vi "fgv_cursor_data.vi"(0 "cursor_idx_set":i32, 1 "plot_data_set":cluster{"array type (2D Dbl)":dbl[], dbl[]}[](array[cluster])=[{"array type (2D Dbl)"=array[301 elements], array[301 elements]}, {"array type (2D Dbl)"=array[301 elements], array[301 elements]}, {"array type (2D Dbl)"=array[301 elements], array[301 elements]}, {"array type (2D Dbl)"=array[301 elements], array[301 elements]}, {"array type (2D Dbl)"=[], []}, {"array type (2D Dbl)"=[], []}, {"array type (2D Dbl)"=[], []}, {"array type (2D Dbl)"=[], []}], 3 "cursor_mode_set":bool, 5 "cursor_pos_set":i32, 7 "cursor_color_set":T1, 9 "mode":string(combo)="Get", 11 "Error in":errorcluster, 12 "plot_id_set":i32) -> (4 "cursor_idx_get":i32, 6 "cursor_pos_get":i32, 8 "cursor_color_get":T1, 10 "cursor_data_get":T2, 13 "plot_id_get":i32, 14 "cursor_mode_get":bool, 15 "error out":errorcluster)   [LabVIEW 2025]
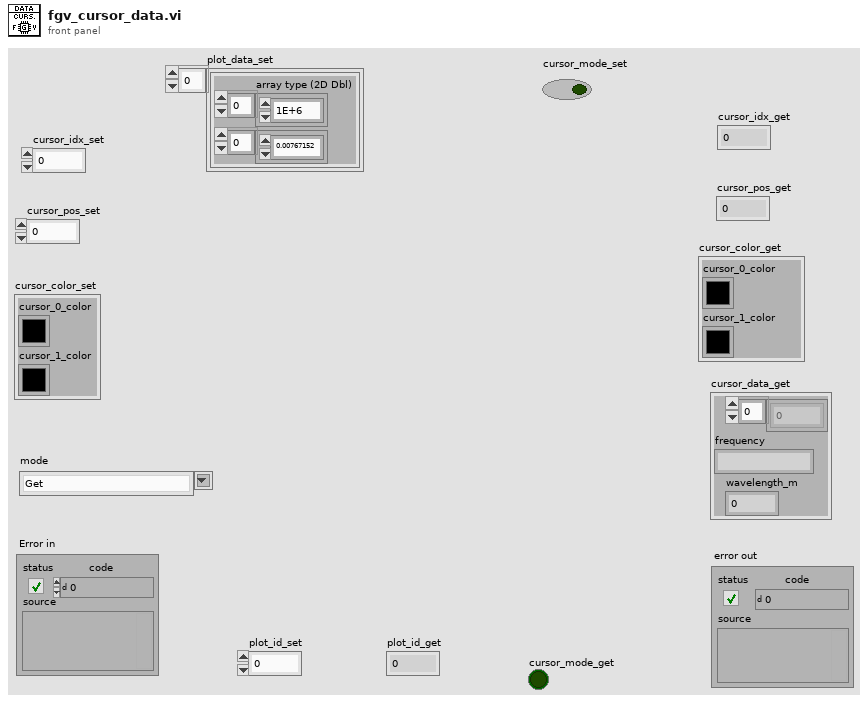
[diagram p1: front panel]
types:
  T1 = cluster{"cursor_0_color":u32, "cursor_1_color":u32}
  T2 = cluster{"cursor_data":dbl[], "frequency":string, "wavelength_m":dbl}
  T3 = cluster{dbl[], "String":string, "wavelength_m":dbl}
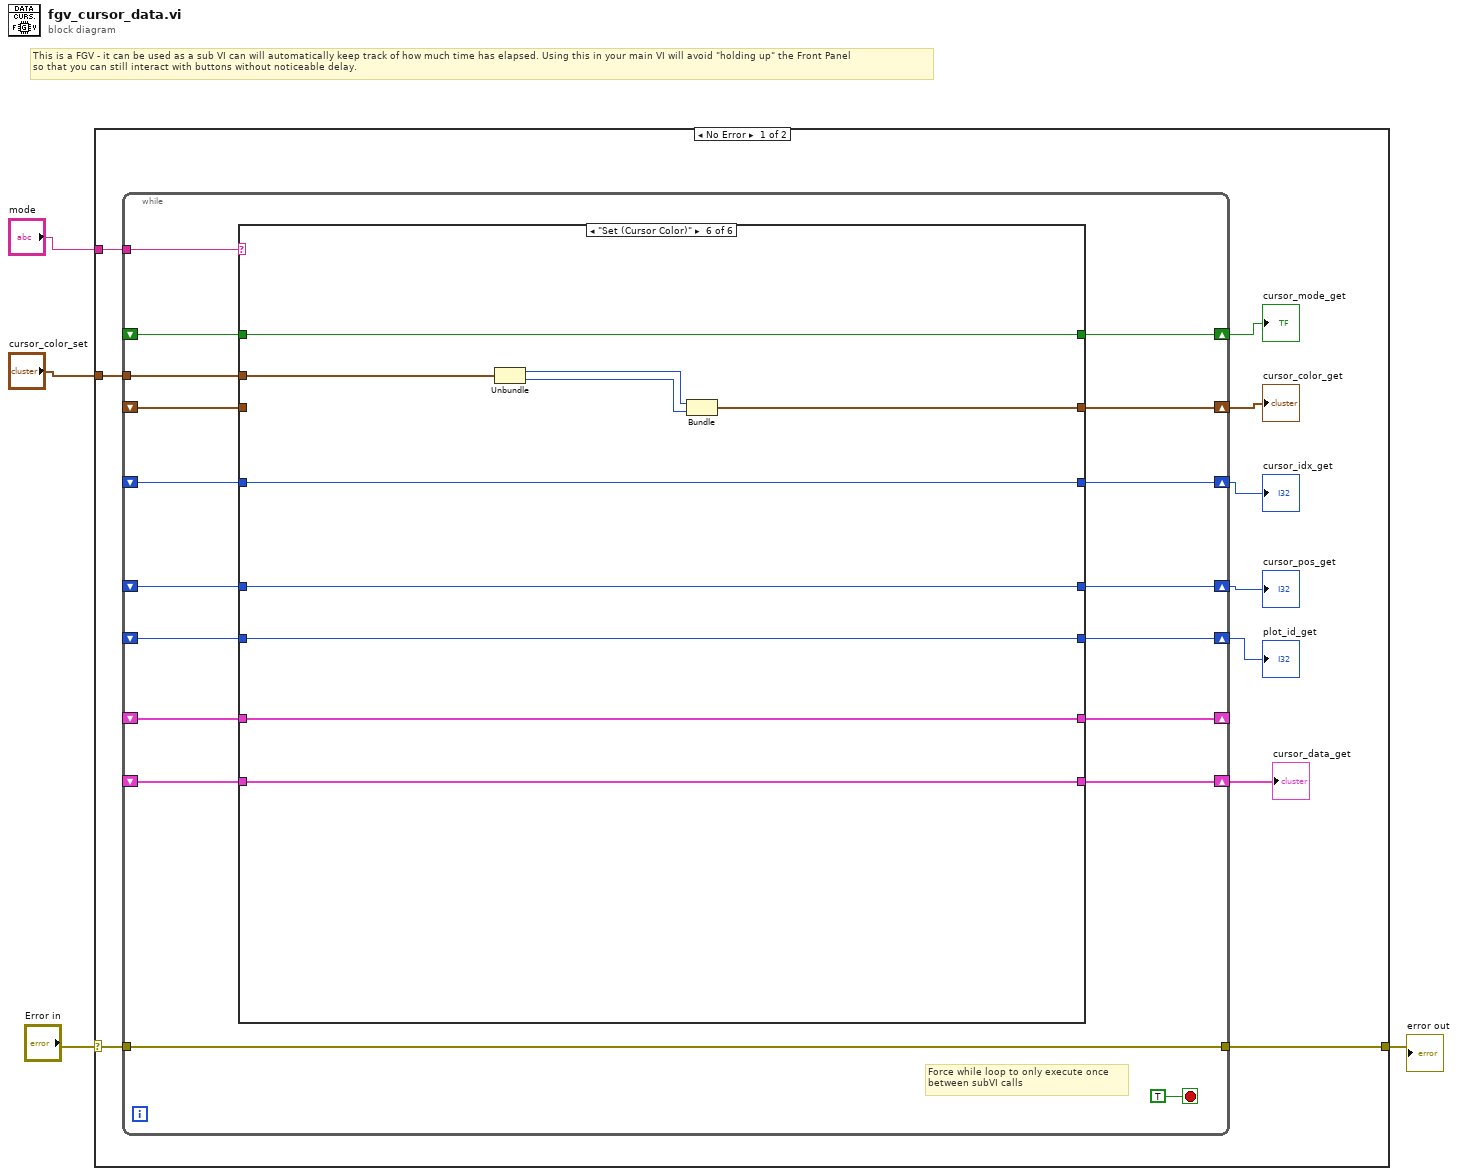
[diagram p0: block diagram]
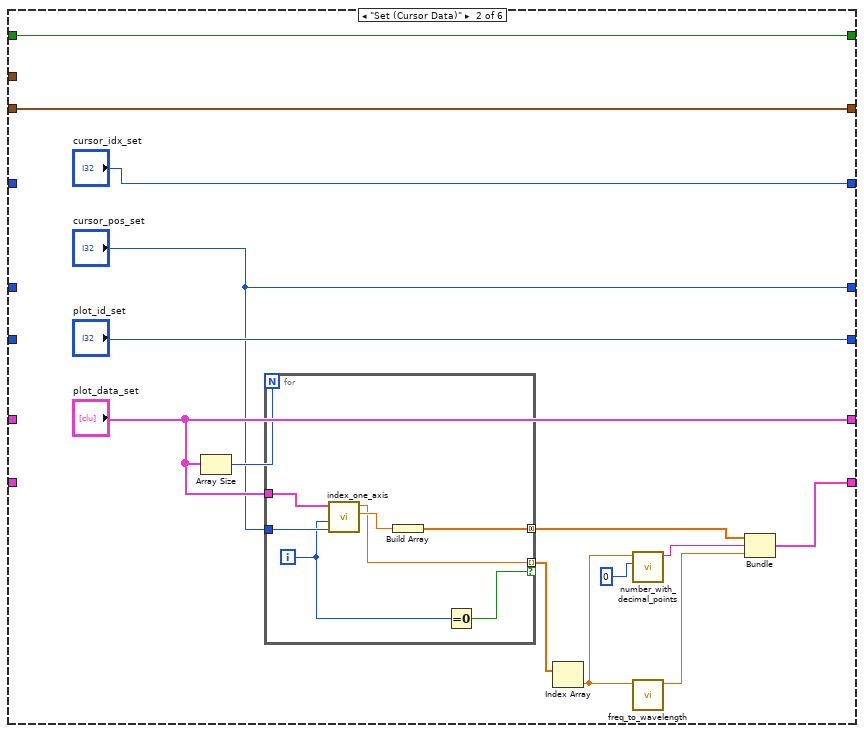
[diagram p3: hidden frame]
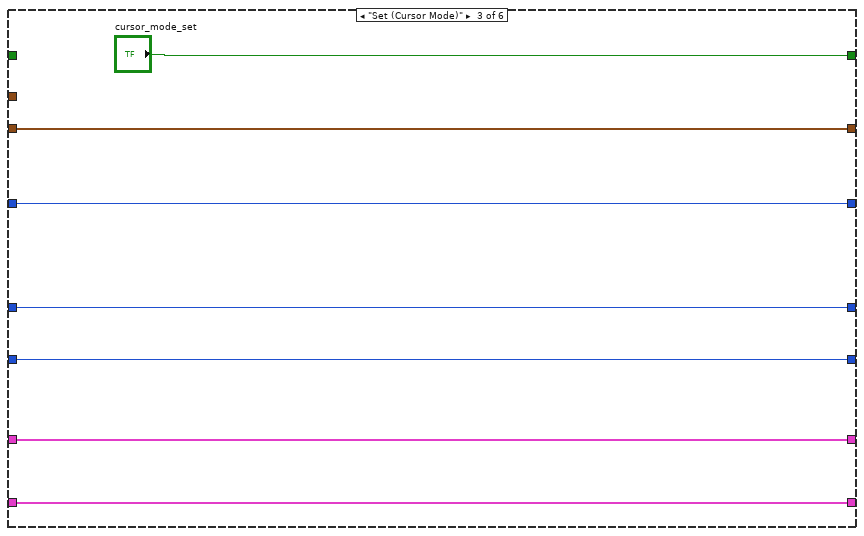
[diagram p4: hidden frame]
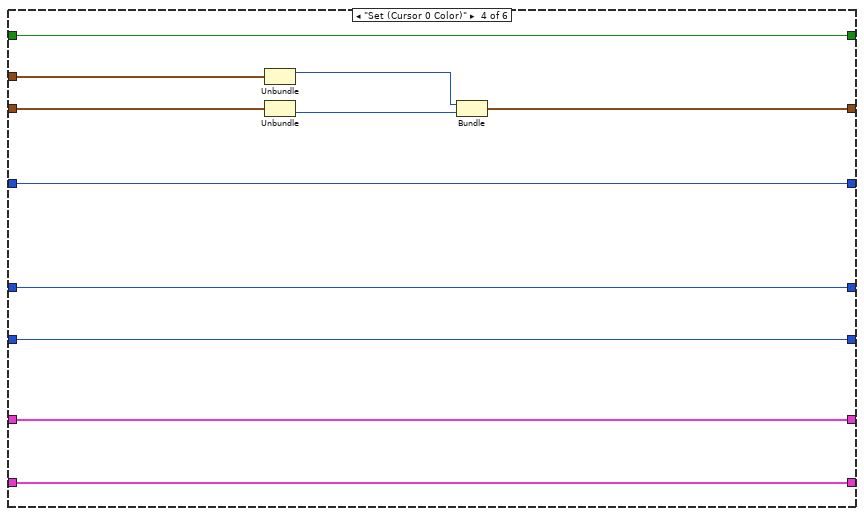
[diagram p5: hidden frame]
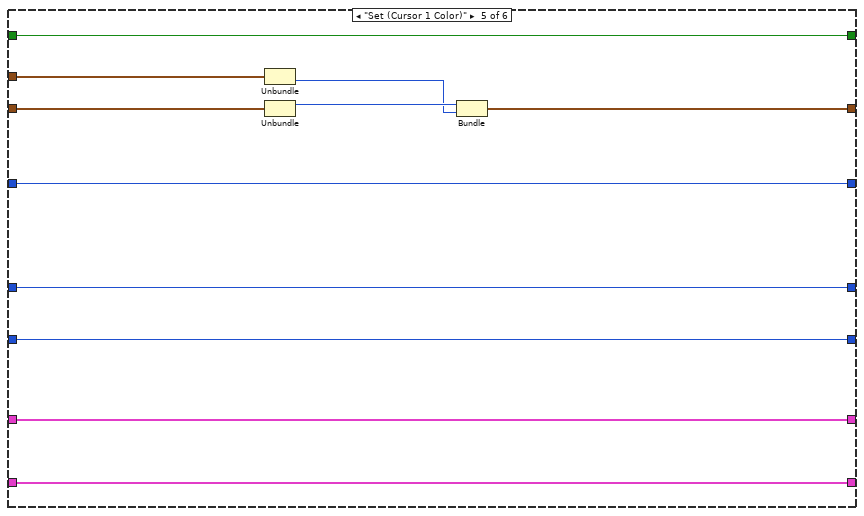
[diagram p6: hidden frame]
diagram:
  # "This is a FGV - it can be used as a sub VI can will automatically keep track of how much time has elapsed. Using this in your main VI will avoid \"holding up\" the Front Panel \nso that you can still interact with buttons without noticeable delay."
  n1 = case shown="No Error" "Error in" {
    selector: "Error in" -> [w14 w100]
    tunnel: [w13 w100] -> w3
    tunnel: "mode" -> [w12 _]
    tunnel: "cursor_color_set" -> [w5 _]
    frame No Error {
      n2 = while {
        shift-right: [w30] -> w10
        shift-left: _ -> [w31]
        tunnel: w14 -> [w29]
        tunnel: [w29] -> w13
        tunnel: w12 -> [w28]
        shift-right: [w27] -> w11
        shift-left: _ -> [w26]
        shift-right: [w25] -> _
        shift-left: _ -> [w24]
        shift-right: [w23] -> w9
        shift-left: _ -> [w22]
        shift-right: [w21] -> w8
        shift-left: _ -> [w20]
        shift-right: [w19] -> w7
        shift-left: _ -> [w18]
        shift-right: [w17] -> w6
        shift-left: _ -> [w16]
        tunnel: w5 -> [w15]
        stop <- TRUE stop-if-true
        # "Force while loop to only execute once\nbetween subVI calls"
        n3 = case shown="\"Set (Cursor Color)\"" w28 {
          tunnel: w31 -> [w39 _ w66 w74 w85 w95]
          tunnel: [w39 "cursor_idx_set" w66 w74 w85 w95] -> w30
          tunnel: [w38 "cursor_pos_set" w65 w75 w86 w96] -> w27
          tunnel: w26 -> [w38 _ w65 w75 w86 w96]
          tunnel: [w37 "plot_data_set" w63 w77 w88 w98] -> w25
          tunnel: w24 -> [w37 _ w63 w77 w88 w98]
          tunnel: [w36 w47 w62 w78 w89 w99] -> w23
          tunnel: w22 -> [w36 _ w62 w78 w89 w99]
          tunnel: [w35 "plot_id_set" w64 w76 w87 w97] -> w21
          tunnel: w20 -> [w35 _ w64 w76 w87 w97]
          tunnel: [w34 w41 "cursor_mode_set" w68 w79 w90] -> w19
          tunnel: w18 -> [w34 w41 _ w68 w79 w90]
          tunnel: [w33 w40 w61 w73 w80 w92] -> w17
          tunnel: w16 -> [w33 w40 w61 w72 w84 _]
          tunnel: w15 -> [_ _ _ w71 w81 w93]
          frame "Get", Default {
          }
          frame "Set (Cursor Data)" {
            n4 = Array Size(array="plot_data_set") -> (size(s)=w45:i32)
            n5 = for {
              N: w45 -> [_]
              tunnel: "plot_data_set" -> [w60]
              tunnel: "cursor_pos_set" -> [w59]
              tunnel: [w57] -> w44 mode=concatenating
              tunnel: [w56] -> w51 mode=indexing if=w55
              i -> [w54]
              n6 = call "index_one_axis.vi"("x_index"=w59, "curve_sel"=w54, "graph_data"=w60) -> ("Y"=w58:dbl, "X"=w56:dbl)  [unwired: 7 in]
              n7 = Build Array(w58) -> (w57:dbl[])
              n8 = Equal To 0?(x=w54) -> (x = 0?=w55:bool)
            }
            n9 = Index Array(array=w51) -> (element=w50:dbl)  [unwired: 1 in]
            n10 = call "number_with_decimal_points.vi"("Precision"=i16 0, "Double"=w50) -> ("String"=w49:string)  [unwired: 5 in]
            n11 = call "freq_to_wavelength.vi"("frequency_hz"=w50) -> ("wavelength_m"=w48:dbl)  [unwired: 10 in]
            n12 = Bundle(w44, "String"=w49, "wavelength_m"=w48) -> (w47:T3)  [unwired: 1 in]
          }
          frame "Set (Cursor Mode)" {
          }
          frame "Set (Cursor 0 Color)" {
            n13 = Unbundle(w71) -> ("cursor_0_color"=w69:u32)  [unwired: 1 out]
            n14 = Unbundle(w72) -> ("cursor_1_color"=w70:u32)  [unwired: 1 out]
            n15 = Bundle("cursor_0_color"=w69, "cursor_1_color"=w70) -> (w73:T1)  [unwired: 1 in]
          }
          frame "Set (Cursor 1 Color)" {
            n16 = Unbundle(w81) -> ("cursor_1_color"=w82:u32)  [unwired: 1 out]
            n17 = Unbundle(w84) -> ("cursor_0_color"=w83:u32)  [unwired: 1 out]
            n18 = Bundle("cursor_0_color"=w83, "cursor_1_color"=w82) -> (w80:T1)  [unwired: 1 in]
          }
          frame "Set (Cursor Color)" {
            n19 = Unbundle(w93) -> ("cursor_0_color"=w91:u32, "cursor_1_color"=w94:u32)
            n20 = Bundle("cursor_0_color"=w91, "cursor_1_color"=w94) -> (w92:T1)  [unwired: 1 in]
          }
        }
      }
      "cursor_pos_get" <- w11
      "cursor_idx_get" <- w10
      "cursor_data_get" <- w9
      "plot_id_get" <- w8
      "cursor_mode_get" <- w7
      "cursor_color_get" <- w6
    }
    frame Error {
      # "Case structure checks for errors - if there's an errorr, do nothing except pass the error back out"
    }
  }
  "error out" <- w3
